vi "ActionVIOnDownload.vi"(5 "System Definition Dir":path, 6 "IP address":string, 7 "Details Ref":refnum<vi>, 8 "error in (no error)":errorcluster, 10 "WebDAV session in":T1, 11 "Device Item Ref in":T2 format="%.0x") -> (0 "error out":errorcluster, 2 "WebDAV session out":T1, 3 "Device Item Ref out":T2 format="%.0x")   [LabVIEW 2020, in "DSF System Explorer.lvlib"]
uses:
  DSF System Explorer.lvlib
  <vilib>/NI VeriStand/Custom Device API/Custom Device Item Ref.ctl
  <vilib>/WebDAVClient/Advanced/SessionHandle.ctl
  DSF Shared.lvlib
  Source/DSF Core.lvlibp
  <vilib>/NI VeriStand/Custom Device API/Custom Device API.lvlib
  <vilib>/WebDAVClient/NI_WebDAV.lvlib
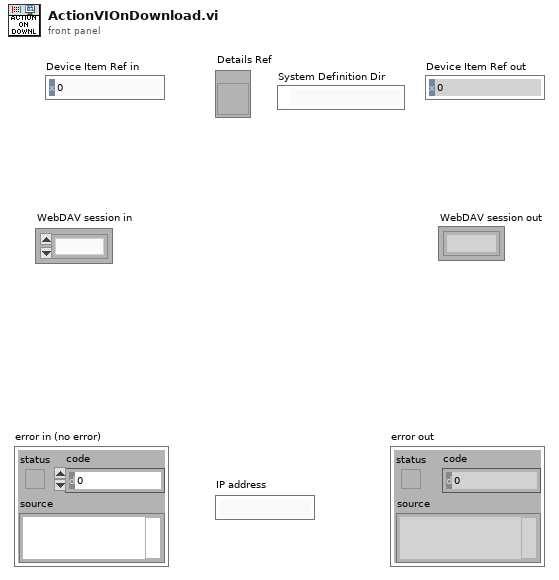
[diagram p1: front panel]
types:
  T1 = typedef "NI_WebDAV.lvlib/SessionHandle.ctl" = refnum<k1>
  T2 = typedef "Custom Device API.lvlib/Custom Device Item Ref.ctl" = u64
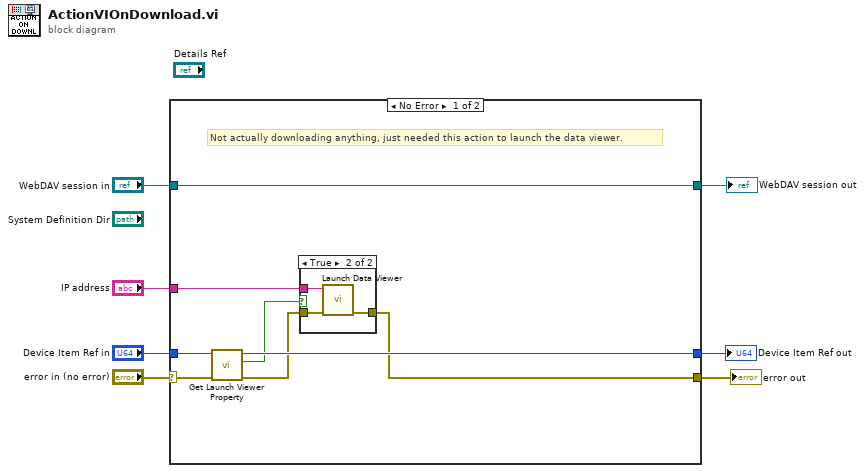
[diagram p0: block diagram]
diagram:
  n1 = case shown="No Error" "error in (no error)" {
    selector: "error in (no error)" -> [w12 w22]
    tunnel: [w9 w22] -> w6
    tunnel: "WebDAV session in" -> [w15 w21]
    tunnel: [w15 w21] -> w2
    tunnel: "Device Item Ref in" -> [w14 w20]
    tunnel: [w13 w20] -> w4
    tunnel: "IP address" -> [w11 _]
    frame No Error {
      # "Not actually downloading anything, just needed this action to launch the data viewer."
      n2 = call "Get Launch Viewer Property.vi"("error in (no error)"=w12, "Item Ref in"=w14) -> ("error out"=w10:errorcluster, "launch viewer"=w8:bool, "Item Ref out"=w13:T2)  [unwired: 7 in]
      n3 = case shown="True" w8 {
        tunnel: w11 -> [_ w19]
        tunnel: w10 -> [w16 w18]
        tunnel: [w16 w17] -> w9
        frame False {
        }
        frame True {
          n4 = call "Launch Data Viewer.vi"("error in (no error)"=w18, "Server IP Address (localhost)"=w19) -> ("error out"=w17:errorcluster)  [unwired: 9 in]
        }
      }
    }
    frame Error {
    }
  }
  "error out" <- w6
  "Device Item Ref out" <- w4
  "WebDAV session out" <- w2
